vi "LBO_Cooling.vi"(6 "LBO Cooling Command:":string="LBOH=0;", 7 "system_power_status":T1, 8 "stop":bool) -> (0 "Aproximate Time":string="Estimated Time: 00:00:00 / 00:00:00", 9 "Battery Life":u8(slide) max=100 step=1 scale=0.0..100.0)   [LabVIEW 2013]
uses:
  <vilib>/Instr/_visa.llb/VISA Configure Serial Port (Instr).vi
  kernel32.dll
panel:
  out "AC Power":bool
  out "DC Power":bool
  out "High":bool
  out "Medium":bool
  out "Critical":bool
  out "Charging":bool
  out "No System Battery":bool
  in  "flow control":u16(ring) items=["None"=0, "XON/XOFF"=1, "RTS/CTS"=2, "DTR/DSR"=4]
  in  "stop bits":u16(ring)=10 items=["1.0"=10, "1.5"=15, "2.0"=20]
  in  "parity":u16(ring) items=["None", "Odd", "Even", "Mark", "Space"]
  in  "data bits":u16=8 min=5 max=8 step=1
  in  "Laser  Serial Connetction:":refnum<visa-resource-name>="COM1"
  in  "baud rate":u32=9600
  # "Please: (1) Restart this VI once in a while;\n           (2) Restart after power outage"
  # "Acquiring Battery Status:"
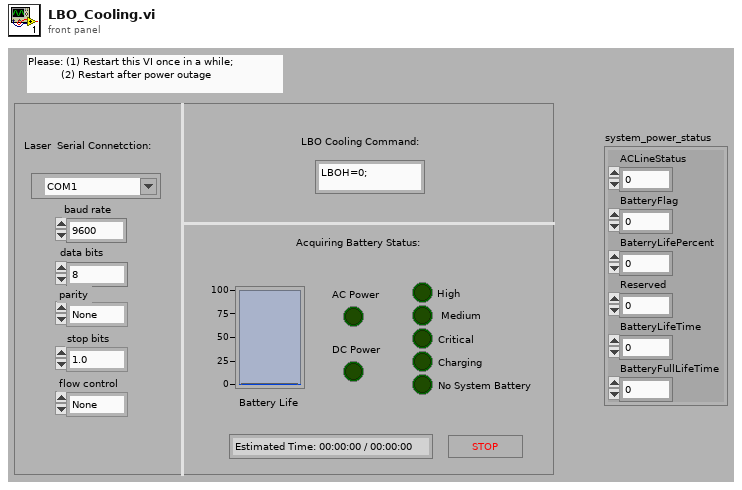
[diagram p1: front panel]
types:
  T1 = cluster{"ACLineStatus":u8, "BatteryFlag":u8, "BaterryLifePercent":u8, "Reserved":u8, "BatteryLifeTime":i32, "BatteryFullLifeTime":i32}
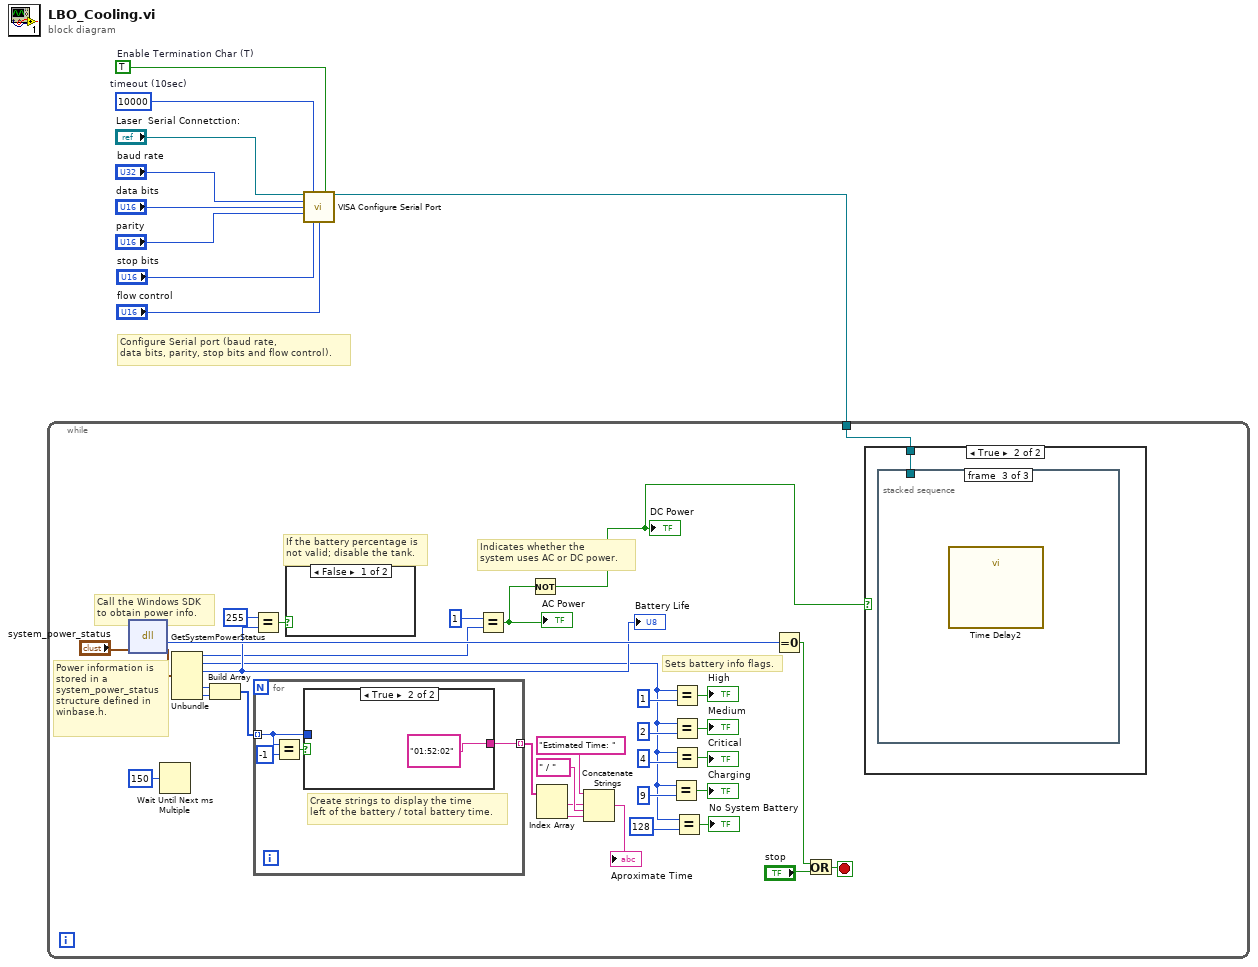
[diagram p0: block diagram]
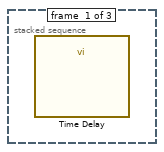
[diagram p3: hidden frame]
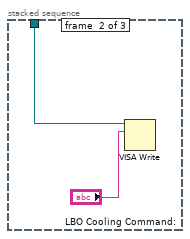
[diagram p4: hidden frame]
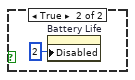
[diagram p5: hidden frame]
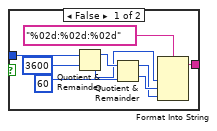
[diagram p6: hidden frame]
diagram:
  w5 = TRUE  # Enable Termination Char (T)
  w6 = u32 10000  # timeout (10sec)
  # "Configure Serial port (baud rate,\ndata bits, parity, stop bits and flow control)."
  n1 = call-poly "VISA Configure Serial Port"("VISA resource name"="Laser  Serial Connetction:", "timeout (10sec)"=w6, "Enable Termination\nChar (T)"=w5, "baud rate (9600)"="baud rate", "data bits (8)"="data bits", "parity (0:none)"="parity", "stop bits (10: 1 bit)"="stop bits", "flow control (0:none)"="flow control") -> ("VISA resource name out"=w1:refnum<visa-resource-name>)  [unwired: 6 in, 1 out]
  n2 = while {
    tunnel: w1 -> [w12]
    stop <- w41 stop-if-true
    # "Power information is\nstored in a\nsystem_power_status\nstructure defined in\nwinbase.h."
    # "Sets battery info flags."
    # "Indicates whether the\nsystem uses AC or DC power."
    # "If the battery percentage is\nnot valid; disable the tank."
    # "Call the Windows SDK\nto obtain power info."
    n3 = dll-call lib="kernel32.dll" fn="GetSystemPowerStatus"("system_power_status"="system_power_status") -> (w42:i32, "system_power_status"=w38:T1)  [unwired: 3 in, 2 out]
    n4 = Wait Until Next ms Multiple(millisecond multiple=u32 150) -> ()  [unwired: 1 out]
    n5 = Unbundle(w38) -> ("ACLineStatus"=w11:u8, "BatteryFlag"=w19:u8, "BaterryLifePercent"=w20:u8, "BatteryLifeTime"=w35:i32, "BatteryFullLifeTime"=w34:i32)  [unwired: 1 out]
    "Battery Life" <- w20
    n6 = Build Array(w35, w34) -> (w33:i32[])
    n7 = Equal?(x=u8 255, y=w20) -> (x = y?=w21:bool)
    n8 = for {
      tunnel: w33 -> [w50] mode=indexing
      tunnel: [w49] -> w13 mode=indexing
      # "Create strings to display the time\nleft of the battery / total battery time."
      n9 = Equal?(x=w50, y=-1) -> (x = y?=w51:bool)
      n10 = case shown="True" w51 {
        tunnel: w50 -> [w58 _]
        tunnel: [w57 "01:52:02"] -> w49
        frame False {
          n11 = Quotient & Remainder(x=w58, y=3600) -> (x-y*floor(x/y)=w56:i32, floor(x/y)=w55:i32)
          n12 = Quotient & Remainder(x=w56, y=60) -> (x-y*floor(x/y)=w53:i32, floor(x/y)=w54:i32)
          n13 = Format Into String(format string="%02d:%02d:%02d", w55, w54, w53) -> (resulting string=w57:string)  [unwired: 2 in, 1 out]
        }
        frame True {
        }
      }
    }
    n14 = case shown="False" w21 {
      frame False {
      }
      frame True {
        n15 = property on="Battery Life" class="Slide (strict)"("Disabled"=u8 2) -> ()  [unwired: 2 in, 2 out]
      }
    }
    n16 = Equal?(x=u8 1 ("y"), y=w11) -> (x = y?=w36:bool)
    "AC Power" <- w36
    n17 = Not(x=w36) -> (.not. x?=w10:bool)
    "DC Power" <- w10
    n18 = Index Array(array=w13) -> (element #1=w14:string, element #2=w17:string)  [unwired: 2 in]
    n19 = Concatenate Strings("Estimated Time: " ("format string"), w14, " / " ("format string"), w17) -> (→"Aproximate Time":string)
    n20 = Equal?(x=w19, y=u8 9) -> (x = y?=→"Charging":bool)
    n21 = Equal?(x=w19, y=u8 1) -> (x = y?=→"High":bool)
    n22 = Equal?(x=w19, y=u8 2) -> (x = y?=→"Medium":bool)
    n23 = Equal?(x=w19, y=u8 4) -> (x = y?=→"Critical":bool)
    n24 = Equal?(x=w19, y=u8 128) -> (x = y?=→"No System Battery":bool)
    n25 = Equal To 0?(x=w42) -> (x = 0?=w39:bool)
    n26 = Or(x=w39, y="stop") -> (x .or. y?=w41:bool)
    n27 = case shown="True" w10 {
      tunnel: w12 -> [_ w45]
      frame False {
      }
      frame True {
        n28 = stacked-sequence {
          tunnel: w45 -> [_ w47 _]
          frame #0 {
            n29 = call "Time Delay"() -> ()  [unwired: 11 in, 1 out]
          }
          frame #1 {
            n30 = VISA Write(VISA resource name=w47, write buffer="LBO Cooling Command:") -> ()  [unwired: 1 in, 3 out]
          }
          frame #2 {
            n31 = call "Time Delay2"() -> ()  [unwired: 11 in, 1 out]
          }
        }
      }
    }
  }
